vi "TCP - Write and Read Array of Synchronous Messages.vi"(8 "error in":errorcluster, 10 "Array of Messages to Send":string[](array[string]), 11 "TCP Network Connection in":refnum<k5>) -> (0 "error out":errorcluster, 2 "Received Message Array":string[](array[string]), 3 "TCP Network Connection out":refnum<k5>)   [LabVIEW 2021]
doc: "Sends an array of TCP messages and listens for the response to each message."
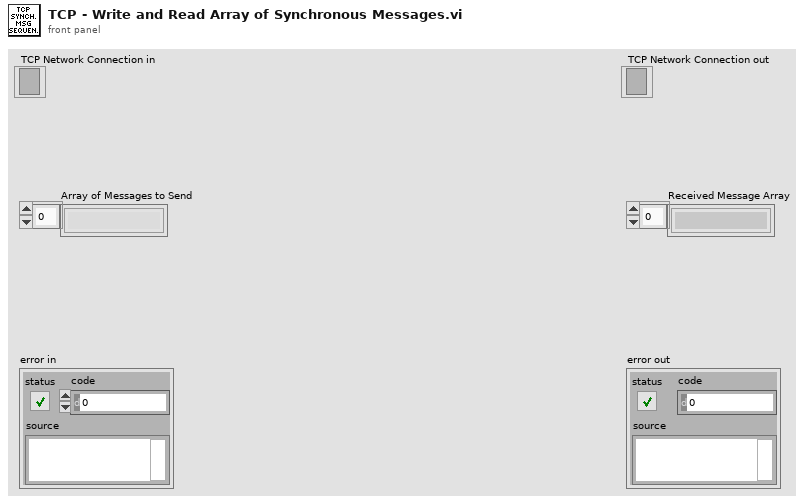
[diagram p1: front panel]
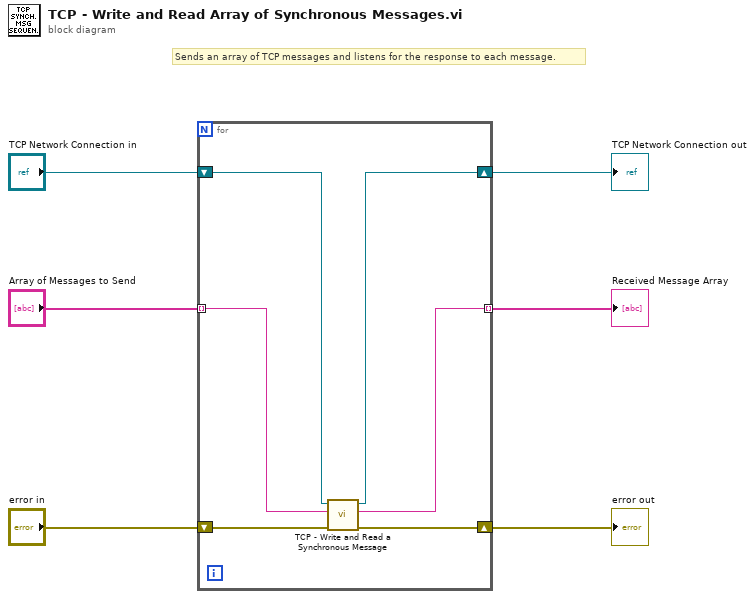
[diagram p0: block diagram]
diagram:
  # "Sends an array of TCP messages and listens for the response to each message."
  n1 = for {
    shift-right: [w11] -> w5
    shift-left: "error in" -> [w12]
    tunnel: "Array of Messages to Send" -> [w10] mode=indexing
    tunnel: [w9] -> w3 mode=indexing
    shift-right: [w7] -> w1
    shift-left: "TCP Network Connection in" -> [w8]
    n2 = call "TCP - Write and Read a Synchronous Message.vi"("error in"=w12, "Message to Send"=w10, "TCP Network Connection in"=w8) -> ("error out"=w11:errorcluster, "Received Text"=w9:string, "TCP Network Connection out"=w7:refnum<k5>)  [unwired: 6 in]
  }
  "TCP Network Connection out" <- w1
  "error out" <- w5
  "Received Message Array" <- w3
